vi "FPGA_DMAOpen.vi"(8 "error in (no error)":errorcluster) -> (0 "error out":errorcluster, 3 "DMADevRef":T1)   [LabVIEW 2017]
uses:
  <vilib>/Rock Robotics/SystemInterfaces/DMA/FPGA_DMADevRef.ctl
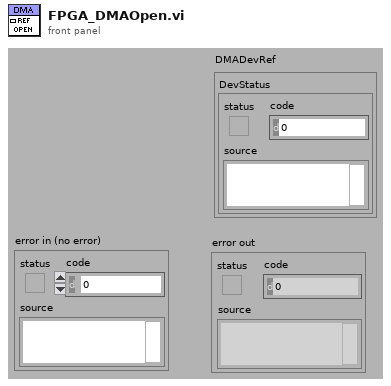
[diagram p1: front panel]
types:
  T1 = typedef "FPGA_DMADevRef.ctl" = cluster{"DevStatus":errorcluster}
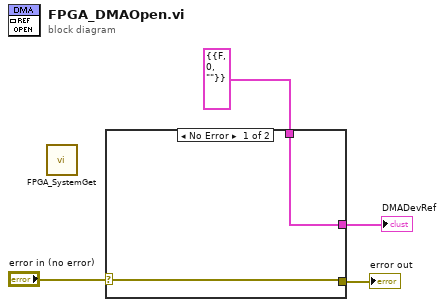
[diagram p0: block diagram]
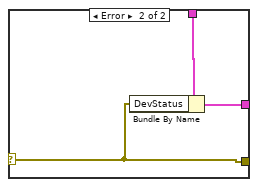
[diagram p2: hidden frame]
diagram:
  n1 = call <vilib>:"FPGA_SystemGet.vi"() -> ()  [unwired: 2 in, 10 out]
  n2 = case shown="No Error" "error in (no error)" {
    selector: "error in (no error)" -> [w5 w7]
    tunnel: T1 {"DevStatus"={"status"=FALSE, "code"=0, "source"=""}} ("DMADevRef") -> [w6 w9]
    tunnel: [w6 w8] -> w1
    tunnel: [w5 w7] -> w3
    frame No Error {
    }
    frame Error {
      n3 = Bundle By Name(cluster=w9, "DevStatus"=w7) -> (w8:T1)
    }
  }
  "error out" <- w3
  "DMADevRef" <- w1
